vi "Get Gyro Angle.vi"(8 "error in":errorcluster) -> (0 "error out":errorcluster, 3 "Gyro Angle":dbl)   [LabVIEW 2016, in "Path Track.lvlib"]
uses:
  Path Track.lvlib
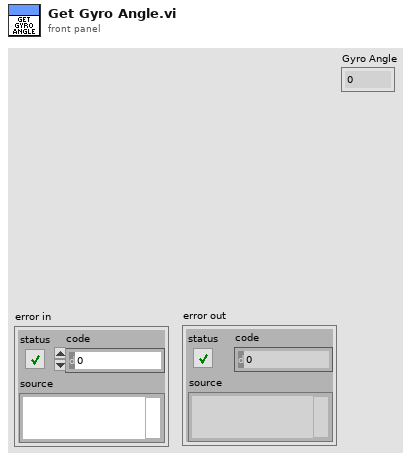
[diagram p1: front panel]
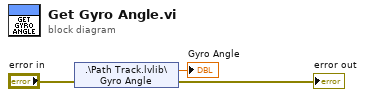
[diagram p0: block diagram]
diagram:
  n1 = shared-variable ".\\Path Track.lvlib\\Gyro Angle"(error in="error in") -> (→"Gyro Angle":dbl, error out=→"error out":errorcluster)
